vi "scan frame to tip.vi"() -> ()   [LabVIEW 2010]
uses:
  <userlib>/Nanonis Prog Interface V5/Nanonis Prog Interface.lvlib
panel:
  in  "Scan Frame":bool
  # "to Tip"
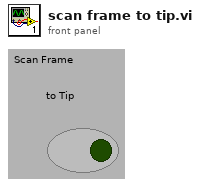
[diagram p1: front panel]
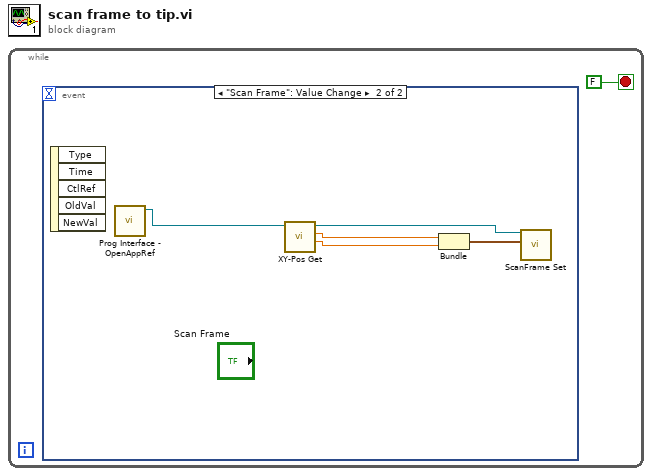
[diagram p0: block diagram]
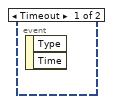
[diagram p2: hidden frame]
diagram:
  n1 = while {
    stop <- FALSE stop-if-true
    n2 = event shown="[1] \"Scan Frame\": Value Change" {
      selector: _ -> [_ _]
      dyn-events: _ -> [_ _]
      timeout: _ -> [_ _]
      event Timeout {
        n3 = event-data() -> ()  [unwired: 1 in, 2 out]
      }
      event "Scan Frame": Value Change {
        n4 = event-data() -> ()  [unwired: 1 in, 5 out]
        n5 = call <userlib>:"Prog Interface - OpenAppRef.vi"() -> ("Application reference"=w5:refnum<vi>)  [unwired: 6 in, 1 out]
        n6 = call <userlib>:"XY-Pos Get.vi"("Application ref in"=w5) -> ("Y (m)"=w3:sgl, "X (m)"=w2:sgl, "Application ref out"=w6:refnum<vi>)  [unwired: 6 in, 1 out]
        n7 = Bundle("X (m)"=w2, "Y (m)"=w3) -> (w4:cluster{"X (m)":sgl, "Y (m)":sgl})  [unwired: 1 in]
        n8 = call <userlib>:"ScanFrame Set.vi"("Application ref in"=w6, "Center coordinates (m)"=w4) -> ()  [unwired: 12 in, 2 out]
      }
    }
  }
